vi "PD_LabVIEW.vi"() -> ()   [LabVIEW 2016]
uses:
  <vilib>/gmath/interp.llb/Create Mesh Grid (2D) (x,y arrays).vi
  <vilib>/gmath/interp.llb/Interpolate 2D (2d X,Y).vi
  <vilib>/gmath/NI_Gmath.lvlib
panel:
  in  "Z":dbl[][](array[numeric])
  out "Intensity Graph":dbl[][](graph)
  in  "Depth 2":i32=2000
  # "INPUT ARRAY SIZE"
  # "POLAR REPRESENTATION OF I/P ARRAY"
  # "CARTESIAN REPRESENTATION OF I/P ARRAY"
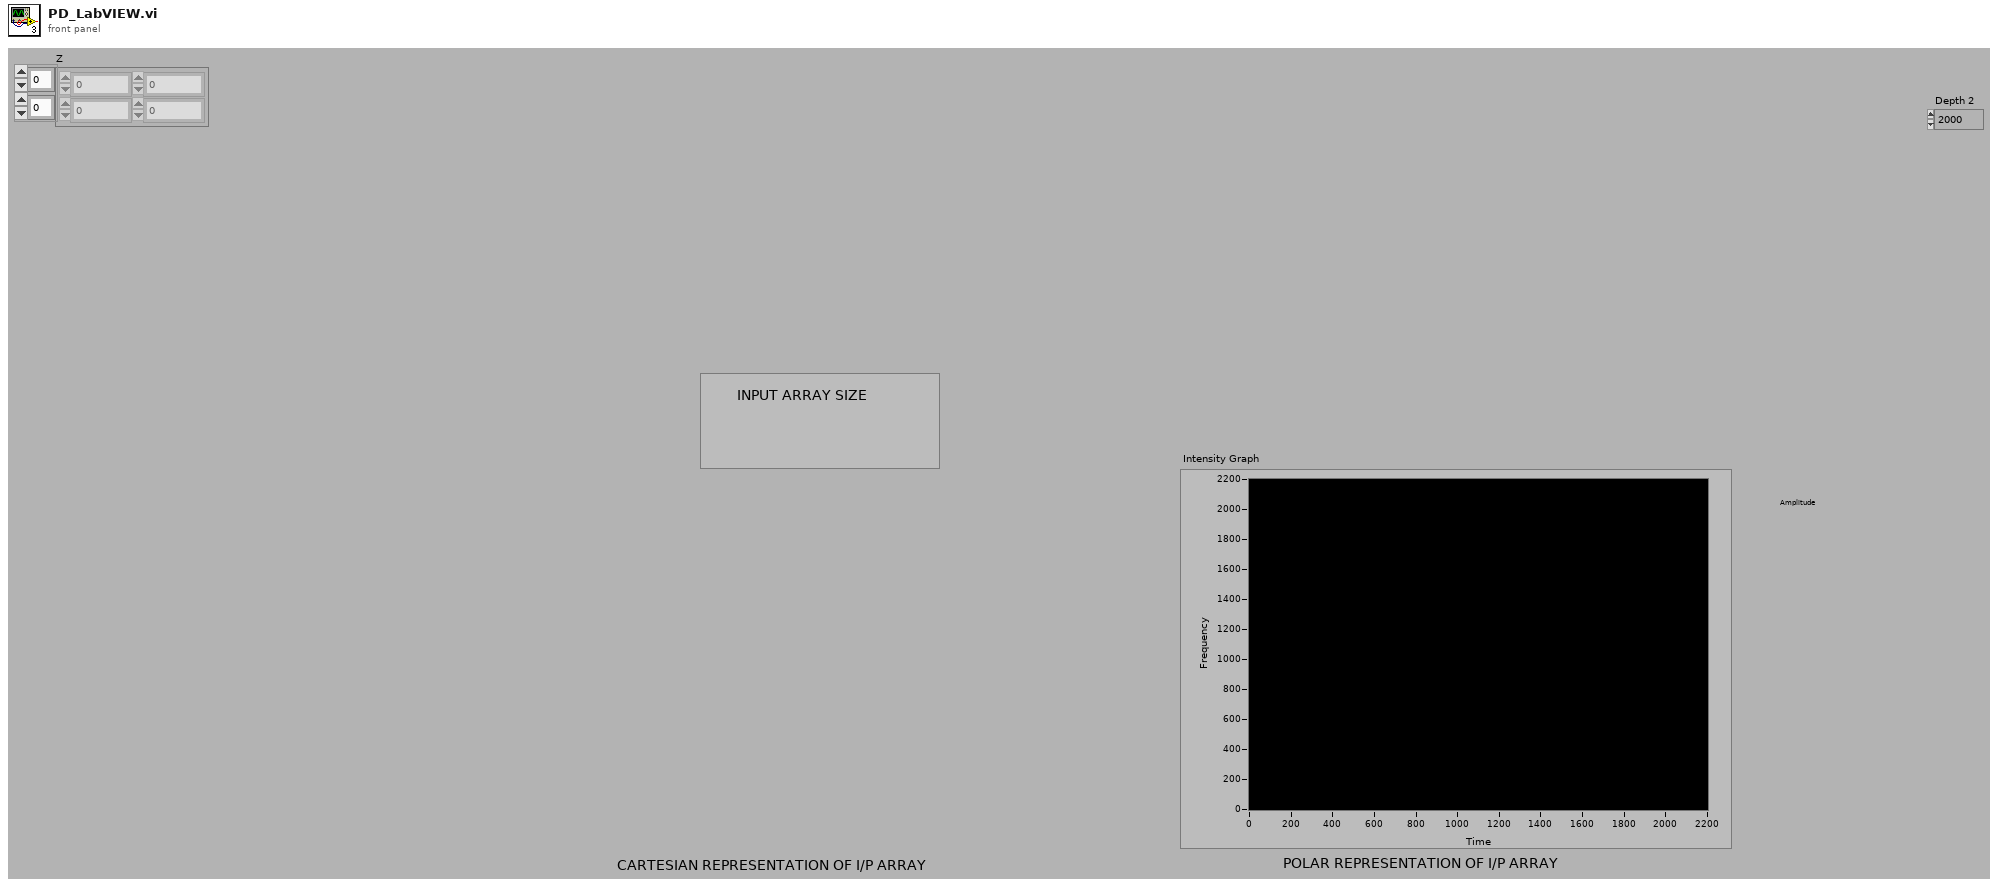
[diagram p1: front panel]
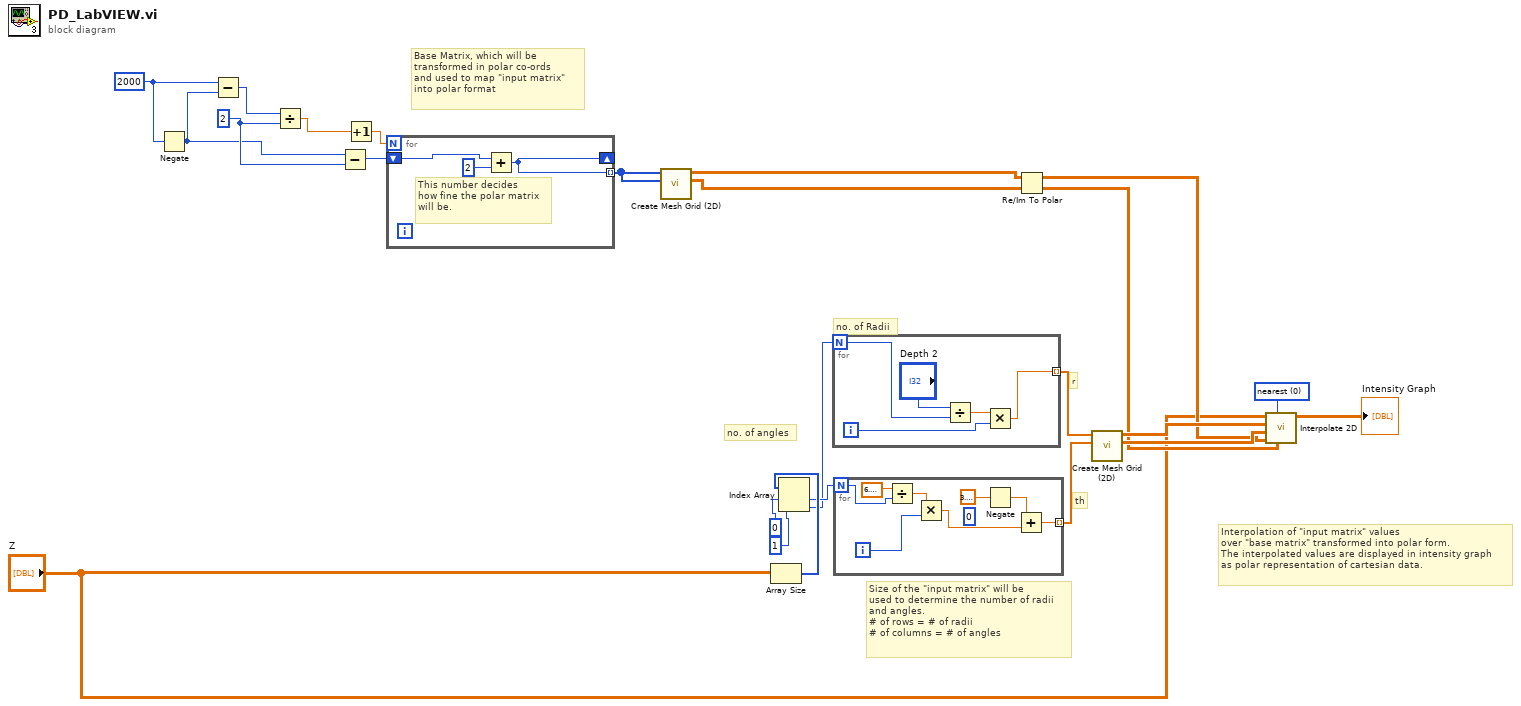
[diagram p0: block diagram]
diagram:
  w2 = 2000 ("x")
  w11 = 0 items=["nearest", "bilinear", "bicubic", "bicubic spline"] ("method")
  w21 = 2 ("y")
  # "Interpolation of \"input matrix\" values\nover \"base matrix\" transformed into polar form.\nThe interpolated values are displayed in intensity graph\nas polar representation of cartesian data."
  # "Size of the \"input matrix\" will be\nused to determine the number of radii\nand angles.  \n# of rows = # of radii\n# of columns = # of angles"
  # "Base Matrix, which will be\ntransformed in polar co-ords\nand used to map \"input matrix\" \ninto polar format"
  # "th"
  # "r"
  # "no. of Radii"
  # "no. of angles"
  n1 = Negate(x=w2) -> (-x=w17:i32)
  n2 = Subtract(x=w2, y=w17) -> (x-y=w22:i32)
  n3 = Divide(x=w22, y=w21) -> (x/y=w19:dbl)
  n4 = Subtract(x=w17, y=w21) -> (x-y=w20:i32)
  n5 = Increment(x=w19) -> (x+1=w18:dbl)
  n6 = for {
    N: w18 -> [_]
    tunnel: [w25] -> w16 mode=indexing
    shift-right: [w25] -> _
    shift-left: w20 -> [w26]
    # "This number decides\nhow fine the polar matrix\nwill be."
    n7 = Add(x=w26, y=2) -> (x+y=w25:i32)
  }
  n8 = call-poly <vilib>:"Create Mesh Grid (2D).vi"("y domain"=w16, "x domain"=w16) -> ("Y"=w23:dbl[][], "X"=w24:dbl[][])  [unwired: 7 in, 1 out]
  n9 = Array Size(array="Z") -> (size(s)=w7:i32[])
  n10 = Index Array(array=w7, index #1=0 ("index"), index #2=1 ("index")) -> (element #1=w4:i32, element #2=w3:i32)
  n11 = for {
    N: w3 -> [w30]
    tunnel: [w28] -> w9 mode=indexing
    i -> [w29]
    n12 = Divide(x="Depth 2", y=w30) -> (x/y=w31:dbl)
    n13 = Multiply(x=w31, y=w29) -> (x*y=w28:dbl)
  }
  n14 = for {
    N: w4 -> [w38]
    tunnel: [w37] -> w8 mode=indexing
    i -> [w40]
    (unwired) 0
    n15 = Divide(x=6.283185307179586, y=w38) -> (x/y=w39:dbl)
    n16 = Multiply(x=w39, y=w40) -> (x*y=w36:dbl)
    n17 = Negate(x=3.141592653589793) -> (-x=w35:dbl)
    n18 = Add(x=w35, y=w36) -> (x+y=w37:dbl)
  }
  n19 = Re/Im To Polar(2:w23, 3:w24) -> (0:w12:dbl[][], 1:w13:dbl[][])
  n20 = call-poly <vilib>:"Create Mesh Grid (2D).vi"("y domain"=w8, "x domain"=w9) -> ("Y"=w14:dbl[][], "X"=w15:dbl[][])  [unwired: 7 in, 1 out]
  n21 = call-poly <vilib>:"Interpolate 2D.vi"("yi"=w12, "method"=w11, "xi"=w13, "Y"=w14, "X"=w15, "Z"="Z") -> ("zi"=→"Intensity Graph":dbl[][])  [unwired: 2 in, 3 out]
